vi "InvertScreenside.vi"(11 "SlideInDirection":T1) -> (3 "Inverted":T1)   [LabVIEW 2019, in "RT_Game.lvlib" / "Game.lvclass"]
uses:
  Game.lvclass
  ScreenSide.ctl
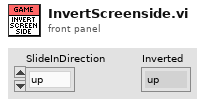
[diagram p1: front panel]
types:
  T1 = typedef "RT_Game.lvlib/Game.lvclass/ScreenSide.ctl" = enum16{"up", "down", "left", "right", "none"}
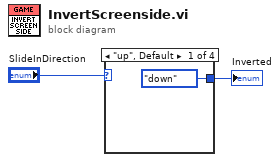
[diagram p0: block diagram]
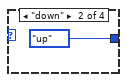
[diagram p2: hidden frame]
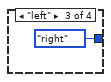
[diagram p3: hidden frame]
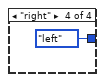
[diagram p4: hidden frame]
diagram:
  n1 = case shown="\"up\", Default" "SlideInDirection" {
    tunnel: [ScreenSide."down" ("SlideDirection(left)") ScreenSide."up" ("SlideDirection(left)") ScreenSide."right" ("SlideDirection(left)") ScreenSide."left" ("SlideDirection(left)")] -> w2
    frame "up", Default {
    }
    frame "down" {
    }
    frame "left" {
    }
    frame "right" {
    }
  }
  "Inverted" <- w2
